vi "GetPlayerStats.vi"(8 "error in (no error)":errorcluster, 11 "ClashRoyale in":refnum<class "StashRoyale.lvclass">) -> (0 "error out":errorcluster, 3 "ClashRoyale out":refnum<class "StashRoyale.lvclass">)   [LabVIEW 2020, in "StashRoyale.lvclass"]
uses:
  StashRoyale.lvclass
  <vilib>/httpClient/LabVIEWHTTPClient.lvlib
  <vilib>/addons/Tools/Unicode/UTF8 Tools.lvlib
  ctl_Player.ctl
  support/JSON.lvlibp
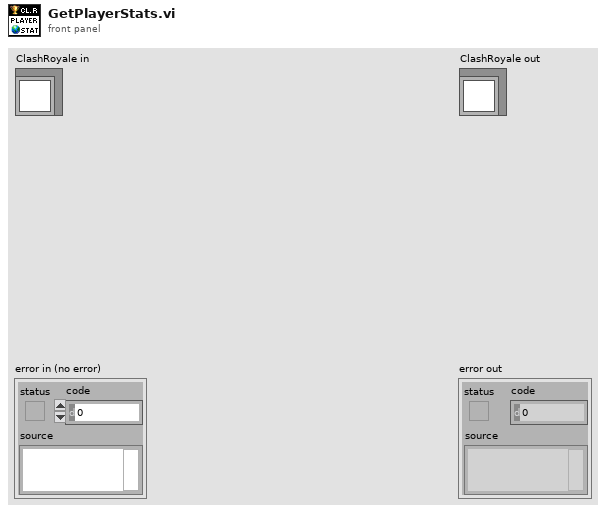
[diagram p1: front panel]
types:
  T1 = typedef "StashRoyale.lvclass/ctl_Player.ctl" = cluster{"name":string, "expLevel":dbl, "trophies":dbl, "bestTrophies":dbl, "wins":dbl, "losses":dbl, "battleCount":dbl, "threeCrownWins":dbl}
  T2 = typedef "LabVIEWHTTPClient.lvlib/ClientHandle.ctl" = refnum<k1>
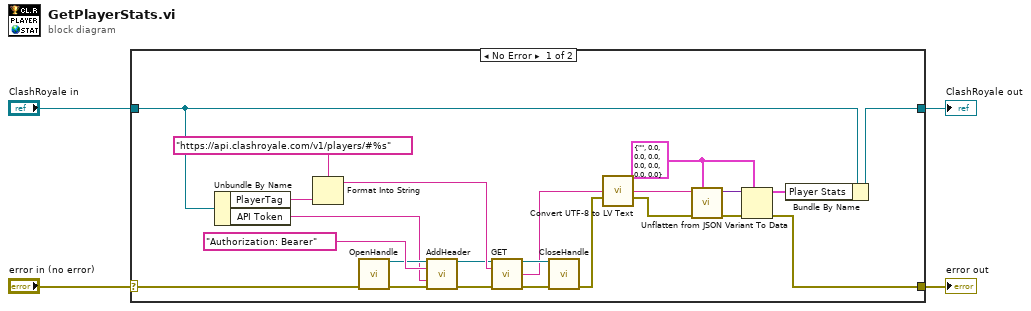
[diagram p0: block diagram]
diagram:
  n1 = case shown="No Error" "error in (no error)" {
    selector: "error in (no error)" -> [w24 w29]
    tunnel: [w5 w29] -> w3
    tunnel: [w19 w28] -> w1
    tunnel: "ClashRoyale in" -> [w21 w28]
    frame No Error {
      w10 = T1 {"name"="", "expLevel"=0.0, "trophies"=0.0, "bestTrophies"=0.0, "wins"=0.0, "losses"=0.0, "battleCount"=0.0, "threeCrownWins"=0.0} ("Player")
      n2 = Unbundle By Name(w21) -> ("PlayerTag"=w20:string, "API Token"=w12:string)
      n3 = Format Into String(format string="https://api.clashroyale.com/v1/players/#%s" ("url"), w20) -> (resulting string=w22:string)  [unwired: 2 in, 1 out]
      n4 = call <vilib>:"OpenHandle.vi"("error in (no error)"=w24) -> ("client handle out"=w16:T2, "error out"=w13:errorcluster)  [unwired: 13 in]
      n5 = call <vilib>:"AddHeader.vi"("client handle"=w16, "header"="Authorization: Bearer", "value"=w12, "error in (no error)"=w13) -> ("client handle out"=w15:T2, "error out"=w14:errorcluster)  [unwired: 10 in]
      n6 = call <vilib>:"GET.vi"("client handle"=w15, "url"=w22, "error in (no error)"=w14) -> ("client handle out"=w27:T2, "body"=w25:string, "error out"=w26:errorcluster)  [unwired: 9 in, 1 out]
      n7 = call <vilib>:"CloseHandle.vi"("client handle"=w27, "error in (no error)"=w26) -> ("error out"=w18:errorcluster)  [unwired: 13 in]
      n8 = call <vilib>:"Convert UTF-8 to LV Text.vi"("UTF-8 Text"=w25, "error in"=w18) -> ("LV Text"=w8:string, "error out"=w6:errorcluster)  [unwired: 12 in]
      n9 = call "Unflatten from JSON.vi"("Type and Defaults"=w10, "error in (no error)"=w6, "JSON String"=w8) -> ("error out"=w7:errorcluster, "data"=w11:variant)  [unwired: 7 in]
      n10 = Variant To Data(error in=w7, type=w10, Variant=w11) -> (data=w9:T1, error out=w5:errorcluster)
      n11 = Bundle By Name(cluster=w21, "Player Stats"=w9) -> (w19:refnum<class "StashRoyale.lvclass">)
    }
    frame Error {
    }
  }
  "error out" <- w3
  "ClashRoyale out" <- w1
